vi "REGB.vi"(2 "D1":bool[](array[boolean]), 3 "R":bool, 4 "C":bool) -> (0 "~Q 2":bool[](array[boolean]), 1 "Q 2":bool[](array[boolean]))   [LabVIEW 2019, in "Triggers.lvlib"]
uses:
  Triggers.lvlib
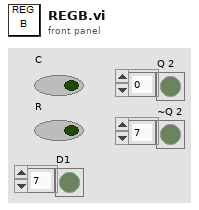
[diagram p1: front panel]
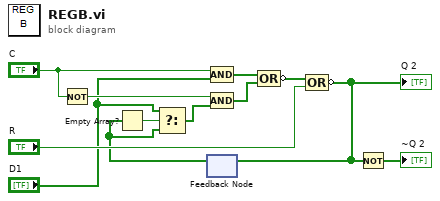
[diagram p0: block diagram]
diagram:
  n1 = Not(x="C") -> (.not. x?=w12:bool)
  n2 = feedback #1() -> (w5:bool[])  [unwired: 1 in]
  n3 = Empty Array?(array=w5) -> (empty?=w8:bool)
  n4 = Select(t="D1", s=w8, f=w5) -> (s? t:f=w4:bool[])
  n5 = Compound Arithmetic op=AND("C", "D1") -> (w11:bool[])
  n6 = Compound Arithmetic op=AND(w12, w4) -> (w10:bool[])
  n7 = Compound Arithmetic op=OR(w11, w10) -> (invert w9:bool[])
  n8 = Compound Arithmetic op=OR(w9, "R") -> (invert w2:bool[])
  "Q 2" <- w2
  n9 = feedback-in #1(w2) -> ()
  n10 = Not(x=w2) -> (.not. x?=→"~Q 2":bool[])
